vi "roof-window-sensor.vi"(7 "LabVIEW Web Service Request":refnum<class "Web Request.lvclass">) -> (3 "roof_window_status":bool)   [LabVIEW 2023]
uses:
  Sensors.vi
  <vilib>/wsapi/Web Request.lvclass
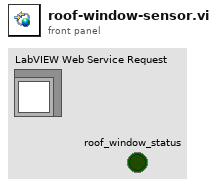
[diagram p1: front panel]
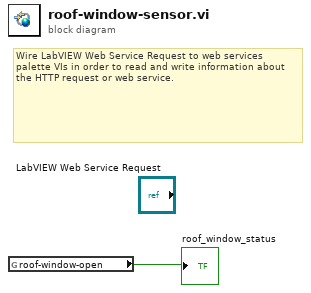
[diagram p0: block diagram]
diagram:
  # "Wire LabVIEW Web Service Request to web services palette VIs in order to read and write information about the HTTP request or web service."
  n1 = global read "Sensors.vi" "roof-window-open"() -> (→"roof_window_status":bool)
